vi "Initialize.vi"(0 "VISA resource name":refnum<visa-resource-name>="GPIB::16", 1 "ID Query? (T: Check)":bool=TRUE, 2 "Reset? (T: Reset)":bool=TRUE, 5 "error in (no error)":errorcluster) -> (14 "VISA resource name out":refnum<visa-resource-name>, 19 "error out":errorcluster)   [LabVIEW 2020, in "Keithley 2100 Series.lvlib"]
doc: "This VI passes the addressing information in the instrument decriptor to the Instr Open VI and returns the instrument ID. You can optionally reset the instrument by setting the front panel reset control. \n\nNote:\nThis Driver is stricly tested with USB."
uses:
  Keithley 2100 Series.lvlib
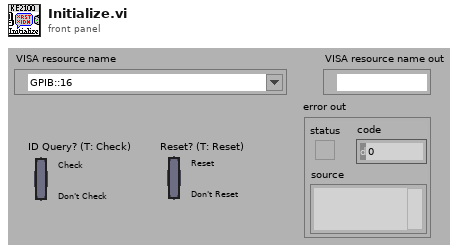
[diagram p1: front panel]
types:
  T1 = cluster{"Status":bool, "Code":i32, "Source (VI Name)":string}
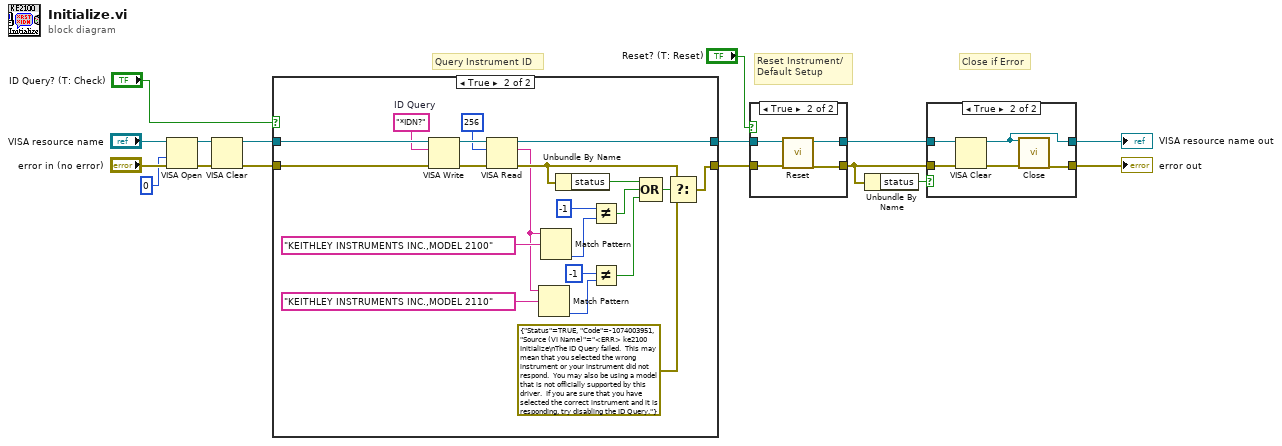
[diagram p0: block diagram]
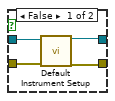
[diagram p3: hidden frame]
diagram:
  # "Close if Error"
  # "Query Instrument ID"
  # "Reset Instrument/\nDefault Setup"
  n1 = VISA Open(access mode=u32 0, error in (no error)="error in (no error)", VISA resource name="VISA resource name") -> (VISA resource name=w2:refnum<visa-resource-name>, error out=w1:errorcluster)  [unwired: 2 in]
  n2 = VISA Clear(VISA resource name=w2, error in (no error)=w1) -> (VISA resource name out=w7:refnum<visa-resource-name>, error out=w6:errorcluster)
  n3 = case shown="True" "ID Query? (T: Check)" {
    tunnel: [w17 w39] -> w15
    tunnel: [w18 w36] -> w16
    tunnel: w7 -> [w18 w37]
    tunnel: w6 -> [w17 w38]
    frame False {
    }
    frame True {
      w29 = "*IDN?"  # ID Query
      n4 = VISA Write(VISA resource name=w37, write buffer=w29, error in (no error)=w38) -> (VISA resource name out=w35:refnum<visa-resource-name>, error out=w33:errorcluster)  [unwired: 1 out]
      n5 = VISA Read(VISA resource name=w35, byte count=u32 256, error in (no error)=w33) -> (VISA resource name out=w36:refnum<visa-resource-name>, read buffer=w19:string, error out=w34:errorcluster)  [unwired: 1 out]
      n6 = Match Pattern(string=w19, regular expression="KEITHLEY INSTRUMENTS INC.,MODEL 2110") -> (offset past match=w25:i32)  [unwired: 1 in, 3 out]
      n7 = Match Pattern(string=w19, regular expression="KEITHLEY INSTRUMENTS INC.,MODEL 2100") -> (offset past match=w31:i32)  [unwired: 1 in, 3 out]
      n8 = Unbundle By Name(w34) -> ("status"=w23:bool)
      n9 = Not Equal?(x=-1, y=w31) -> (x != y?=w22:bool)
      n10 = Not Equal?(x=-1, y=w25) -> (x != y?=w20:bool)
      n11 = Compound Arithmetic op=OR(w23, w22, w20) -> (w21:bool)
      n12 = Select(t=w34, s=w21, f=T1 {"Status"=TRUE, "Code"=-1074003951, "Source (VI Name)"="<ERR> ke2100 Initialize\nThe ID Query failed.  This may mean that you selected the wrong instrument or your instrument did not respond.  You may also be using a model that is not officially supported by this driver.  If you are sure that you have selected the correct instrument and it is responding, try disabling the ID Query."}) -> (s? t:f=w39:T1)
    }
  }
  n13 = case shown="True" "Reset? (T: Reset)" {
    tunnel: w15 -> [w40 w44]
    tunnel: [w41 w47] -> w4
    tunnel: w16 -> [w43 w45]
    tunnel: [w42 w46] -> w12
    frame False {
      n14 = call "Default Instrument Setup.vi"("VISA resource name"=w43, "error in (no error)"=w40) -> ("VISA resource name out"=w42:refnum<visa-resource-name>, "error out"=w41:errorcluster)  [unwired: 16 in]
    }
    frame True {
      n15 = call "Reset.vi"("VISA resource name"=w45, "error in (no error)"=w44) -> ("VISA resource name out"=w46:refnum<visa-resource-name>, "error out"=w47:errorcluster)  [unwired: 16 in]
    }
  }
  n16 = Unbundle By Name(w4) -> ("status"=w3:bool)
  n17 = case shown="True" w3 {
    tunnel: w12 -> [w49 w53]
    tunnel: [w49 w52] -> w11
    tunnel: [w48 w54] -> w10
    tunnel: w4 -> [w48 w51]
    frame False {
    }
    frame True {
      n18 = VISA Clear(VISA resource name=w53, error in (no error)=w51) -> (VISA resource name out=w52:refnum<visa-resource-name>, error out=w50:errorcluster)
      n19 = call "Close.vi"("VISA resource name"=w52, "error in (no error)"=w50) -> ("error out"=w54:errorcluster)  [unwired: 17 in]
    }
  }
  "VISA resource name out" <- w11
  "error out" <- w10
